vi "MainGUI.vi"(8 "ErrorIn":errorcluster, 11 "DotNETCamIn":refnum<class "DotNETCam.lvclass">) -> ()   [LabVIEW 2021, in "DotNETCam.lvclass"]
uses:
  DotNETCam.lvclass
  C:/Localdata/Projects/TriekselSoft/TriekselsoftApplicationFramework/Source/.Externals/Library_YAF/YActor/YActor.lvclass
  DotNETCam_UiCallBackEvents.ctl
  DotNETCam_ClassCast.vi
  .Externals/Library_YAF/YActor/YActor.lvclass
panel:
  in  "Boolean":bool
  out "L_busy":i32
  in  "Exit":bool
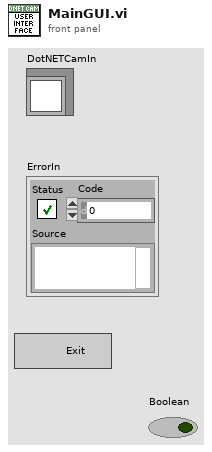
[diagram p1: front panel]
types:
  T1 = typedef "DotNETCam.lvclass/DotNETCam_UiCallBackEvents.ctl" = enum16{"Default", "PersistentDataUpdated", "Worker 1: Do Something"}
  T2 = cluster{"Event":string, "This":refnum<class>, "Data":variant}
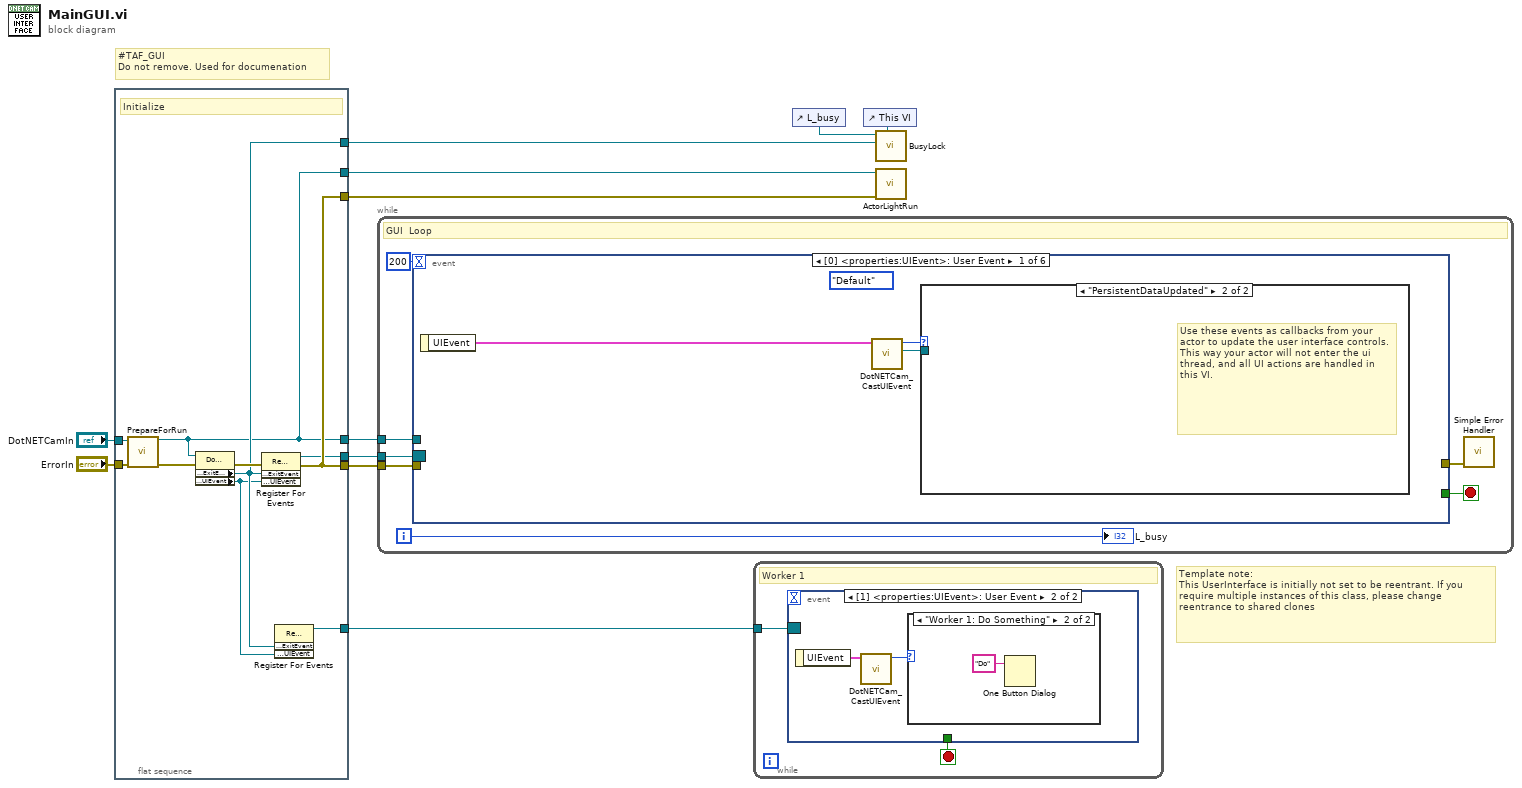
[diagram p0: block diagram]
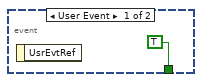
[diagram p2: hidden frame]
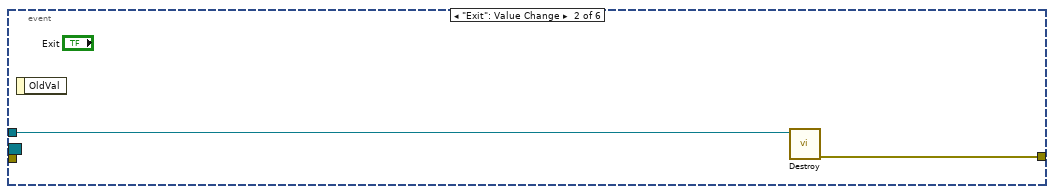
[diagram p5: hidden frame]
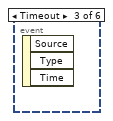
[diagram p6: hidden frame]
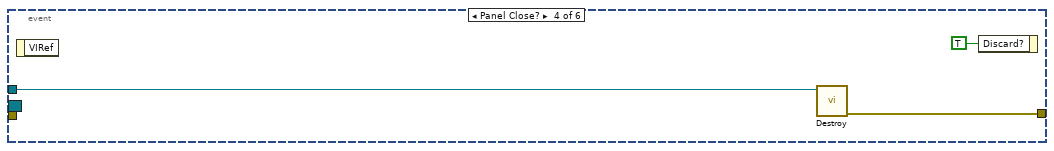
[diagram p7: hidden frame]
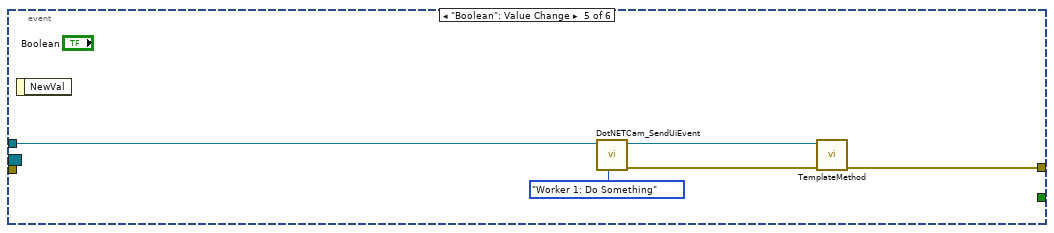
[diagram p8: hidden frame]
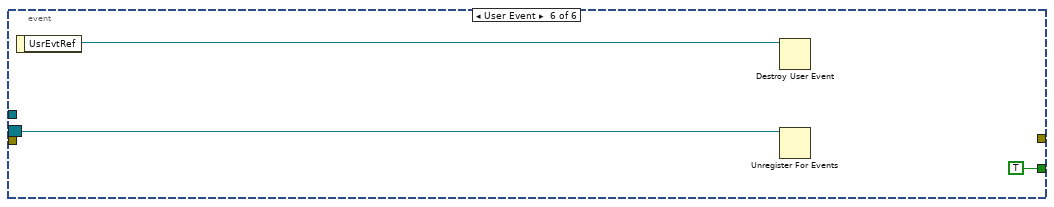
[diagram p9: hidden frame]
diagram:
  # "#TAF_GUI\nDo not remove. Used for documenation"
  # "Template note:\nThis UserInterface is initially not set to be reentrant. If you require multiple instances of this class, please change reentrance to shared clones"
  n1 = flat-sequence {
    tunnel: "ErrorIn" -> [w21]
    tunnel: "DotNETCamIn" -> [w17]
    tunnel: [w16] -> w7
    tunnel: [w15] -> w6
    tunnel: [w14] -> w3
    tunnel: [w12] -> w2
    tunnel: [w18] -> w10
    tunnel: [w12] -> w1
    tunnel: [w18] -> w9
    frame #0 {
      # "Initialize"
      n2 = call-dynamic "PrepareForRun.vi"("ErrorIn"=w21, "YActorIn"=w17) -> ("ErrorOut"=w19:errorcluster, "YActorOut"=w12:refnum<class "DotNETCam.lvclass">)  [unwired: 8 in]
      n3 = property class="DotNETCam"(reference=w12, error in=w19) -> (error out=w20:errorcluster, "properties:ExitEvent"=w14:refnum<user-event>, "properties:UIEvent"=w13:refnum<user-event>)  [unwired: 1 out]
      n4 = register-events(error in=w20, w14, w13) -> (reference out=w16:refnum<event-registration>, error out=w18:errorcluster)  [unwired: 1 in]
      n5 = register-events(w14, w13) -> (reference out=w15:refnum<event-registration>)  [unwired: 2 in, 1 out]
    }
  }
  n6 = while {
    tunnel: w10 -> [w28]
    tunnel: w7 -> [w25]
    tunnel: w2 -> [w22]
    i -> [w24]
    stop <- w26 stop-if-true
    # "GUI  Loop"
    n7 = event shown="[0] <properties:UIEvent>: User Event" {
      selector: w25 -> [_ _ _ _ _ w43]
      dyn-events: _ -> [_ _ _ _ _ _]
      timeout: 200 -> [_ _ _ _ _ _]
      tunnel: w28 -> [_ _ _ _ _ _]
      tunnel: [_ _ _ _ _ TRUE] -> w26
      tunnel: [_ w33 _ w36 w41 _] -> w27
      tunnel: w22 -> [_ w32 _ w34 w39 _]
      event User Event {
        (unwired) DotNETCam_UiCallBackEvents."Default" ("UiEventNames")
        n8 = event-data() -> ("UIEvent"=w31:T2)  [unwired: 1 in]
        n9 = call "DotNETCam_CastUIEvent.vi"("UIEvent"=w31) -> ("ApplicationGUIOut"=w29:refnum<class "DotNETCam.lvclass">, "UiEventNames"=w30:T1)  [unwired: 8 in, 1 out]
        n10 = case shown="\"PersistentDataUpdated\"" w30 {
          tunnel: w29 -> [_ _]
          frame Default {
          }
          frame "PersistentDataUpdated" {
            # "Use these events as callbacks from your actor to update the user interface controls. This way your actor will not enter the ui thread, and all UI actions are handled in this VI."
          }
        }
      }
      event "Exit": Value Change {
        n11 = event-data() -> ()  [unwired: 1 in, 1 out]
        n12 = call-dynamic "Destroy.vi"("ObjectIn"=w32) -> ("ErrorOut"=w33:errorcluster)  [unwired: 9 in, 1 out]
      }
      event Timeout {
        n13 = event-data() -> ()  [unwired: 1 in, 3 out]
      }
      event Panel Close? {
        n14 = event-data() -> ()  [unwired: 1 in, 1 out]
        n15 = call-dynamic "Destroy.vi"("ObjectIn"=w34) -> ("ErrorOut"=w36:errorcluster)  [unwired: 9 in, 1 out]
        n16 = event-data("Discard?"=TRUE) -> ()  [unwired: 1 in, 1 out]
      }
      event "Boolean": Value Change {
        n17 = event-data() -> ()  [unwired: 1 in, 1 out]
        n18 = call "DotNETCam_SendUiEvent.vi"("UiEventNames"=DotNETCam_UiCallBackEvents."Worker 1: Do Something", "DotNETCamIn"=w39) -> ("ErrorOut"=w40:errorcluster, "DotNETCamOut"=w38:refnum<class "DotNETCam.lvclass">)  [unwired: 8 in]
        n19 = call-dynamic "TemplateMethod.vi"("ErrorIn"=w40, "DotNETCamIn"=w38) -> ("ErrorOut"=w41:errorcluster)  [unwired: 7 in, 2 out]
      }
      event User Event {
        n20 = event-data() -> ("UsrEvtRef"=w42:refnum<user-event>)  [unwired: 1 in]
        n21 = Destroy User Event(user event=w42) -> ()  [unwired: 1 in, 1 out]
        n22 = Unregister For Events(event registration refnum=w43) -> ()  [unwired: 1 in, 1 out]
      }
    }
    n23 = call <vilib>:"Simple Error Handler.vi"("error in (no error)"=w27) -> ()  [unwired: 4 in, 5 out]
    "L_busy" <- w24
  }
  n24 = while {
    tunnel: w6 -> [w46]
    stop <- w45 stop-if-true
    # "Worker 1"
    n25 = event shown="[1] <properties:UIEvent>: User Event" {
      selector: w46 -> [_ _]
      dyn-events: _ -> [_ _]
      timeout: _ -> [_ _]
      tunnel: [TRUE _] -> w45
      event User Event {
        n26 = event-data() -> ()  [unwired: 1 in, 1 out]
      }
      event User Event {
        n27 = event-data() -> ("UIEvent"=w49:T2)  [unwired: 1 in]
        n28 = call "DotNETCam_CastUIEvent.vi"("UIEvent"=w49) -> ("UiEventNames"=w48:T1)  [unwired: 8 in, 2 out]
        n29 = case shown="\"Worker 1: Do Something\"" w48 {
          frame Default {
          }
          frame "Worker 1: Do Something" {
            n30 = One Button Dialog(message="Do") -> ()  [unwired: 1 in, 1 out]
          }
        }
      }
    }
  }
  n31 = control-ref of="L_busy"() -> (w5:refnum<vi>)
  n32 = control-ref of="This VI"() -> (w4:refnum<vi>)
  n33 = call "BusyLock.vi"("BusyLock"=w4, "ExitEvent"=w3, "Counter"=w5) -> ()  [unwired: 9 in]
  n34 = call "ActorLightRun.vi"("ErrorIn"=w9, "YActorIn"=w1) -> ()  [unwired: 8 in, 2 out]
